vi "cDAQ Close.vi"(8 "Error In":errorcluster, 10 "AI Task":refnum<k21>, 11 "Temp Task":refnum<k21>) -> (0 "Error Out":errorcluster)   [LabVIEW 2014]
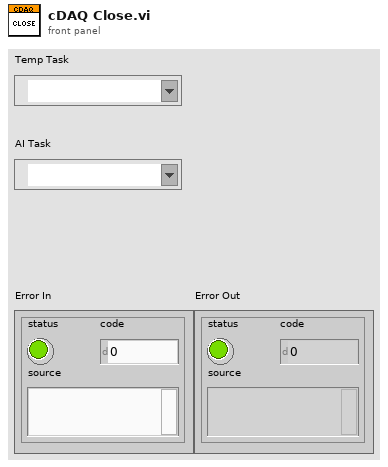
[diagram p1: front panel]
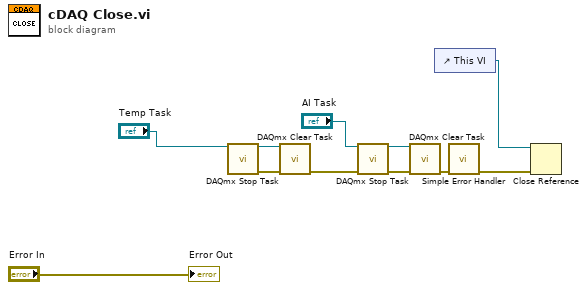
[diagram p0: block diagram]
diagram:
  n1 = call <vilib>:"DAQmx Stop Task.vi"("task/channels in"="Temp Task") -> ("task out"=w4:refnum<k21>, "error out"=w5:errorcluster)  [unwired: 13 in]
  n2 = call <vilib>:"DAQmx Clear Task.vi"("task in"=w4, "error in"=w5) -> ("error out"=w3:errorcluster)  [unwired: 13 in]
  n3 = call <vilib>:"DAQmx Stop Task.vi"("task/channels in"="AI Task", "error in"=w3) -> ("task out"=w6:refnum<k21>, "error out"=w7:errorcluster)  [unwired: 12 in]
  n4 = call <vilib>:"DAQmx Clear Task.vi"("task in"=w6, "error in"=w7) -> ("error out"=w8:errorcluster)  [unwired: 13 in]
  n5 = control-ref of="This VI"() -> (w10:refnum<vi>)
  n6 = call <vilib>:"Simple Error Handler.vi"("error in (no error)"=w8) -> ("error out"=w9:errorcluster)  [unwired: 4 in, 4 out]
  n7 = Close Reference(reference=w10, error in (no error)=w9) -> ()  [unwired: 1 out]
  "Error Out" <- "Error In"
